vi "SynologyWriteRT.vi"() -> ()   [LabVIEW 2018]
panel:
  out "error out":errorcluster
  in  "text":string
  in  "file path (use dialog)":path
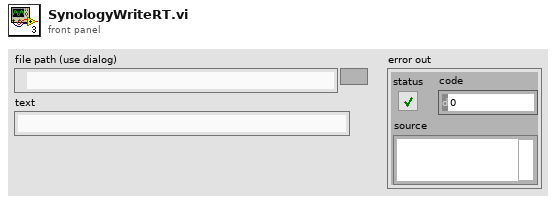
[diagram p1: front panel]
types:
  T1 = enum16{"open", "replace", "create", "open or create", "replace or create", "replace or create with confirmation"}
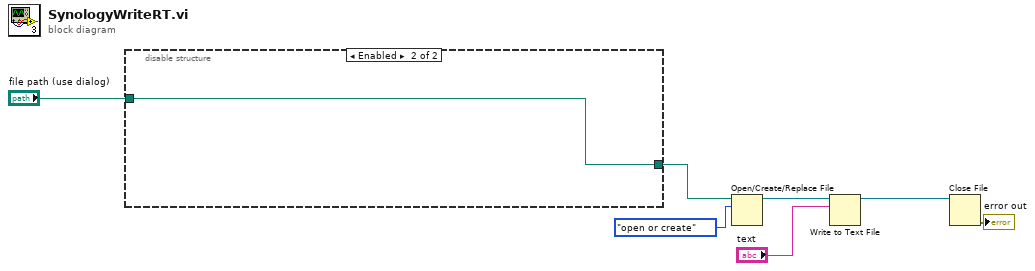
[diagram p0: block diagram]
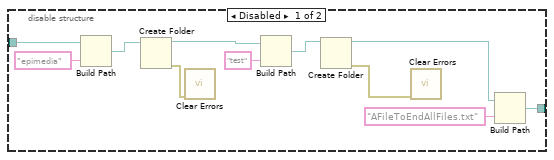
[diagram p2: hidden frame]
diagram:
  n1 = disable-structure shown="Enabled" {
    disable-tunnel: "file path (use dialog)" -> [w18 w19]
    disable-tunnel: [w8 w19] -> w2
    frame Disabled {
      n2 = Build Path(base path=w18, name or relative path="epimedia") -> (appended path=w17:path)
      n3 = Create Folder(path (use dialog)=w17) -> (created path=w14:path, error out=w12:errorcluster)  [unwired: 2 in, 1 out]
      n4 = call <vilib>:"Clear Errors.vi"("error in (no error)"=w12) -> ()  [unwired: 5 in, 2 out]
      n5 = Build Path(base path=w14, name or relative path="test") -> (appended path=w13:path)
      n6 = Create Folder(path (use dialog)=w13) -> (created path=w10:path, error out=w11:errorcluster)  [unwired: 2 in, 1 out]
      n7 = call <vilib>:"Clear Errors.vi"("error in (no error)"=w11) -> ()  [unwired: 5 in, 2 out]
      n8 = Build Path(base path=w10, name or relative path="AFileToEndAllFiles.txt") -> (appended path=w8:path)
    }
    frame Enabled {
    }
  }
  n9 = Open/Create/Replace File(file path (use dialog)=w2, operation (0:open)=T1."open or create") -> (refnum out=w7:refnum<file>)  [unwired: 4 in, 2 out]
  n10 = Write to Text File(file (use dialog)=w7, text="text") -> (refnum out=w6:refnum<file>)  [unwired: 2 in, 2 out]
  n11 = Close File(refnum=w6) -> (error out=→"error out":errorcluster)  [unwired: 1 in, 1 out]
